vi "Error - Fire.vi"(8 "error in (no error)":errorcluster, 9 "Data":variant, 10 "Error Level":T6, 11 "View Model":T1) -> (0 "error out":errorcluster, 3 "View Model":T1)   [LabVIEW 2017]
doc: "Generates Error user event with parameters: Error Level, Error Data."
uses:
  View Model/Controls/View Model.ctl
  View Model/Controls/Shared Model.ctl
  Controls/Error Model.ctl
  Controls/Error Data.ctl
  Controls/Error Level.ctl
  Configuration/Controls/Config Model.ctl
  Configuration/Controls/Config Record.ctl
  Configuration/Controls/Config Data.ctl
  Configuration/Controls/Config Command.ctl
  Controller/Controls/Controler Model.ctl
  Views/Entry Console View/Controls/Entry Console - Wash Steps.ctl
  Controller/Controls/Controller - Overhead.ctl
  Controller/Controls/Controller - States.ctl
  Controller/Controls/Controller - Wash Step.ctl
  Views/Vehicle Position View/Controls/Vehicle - Station Enum.ctl
  Controller/Controls/Controller - Event.ctl
  Controller/Controls/Controller - Commands.ctl
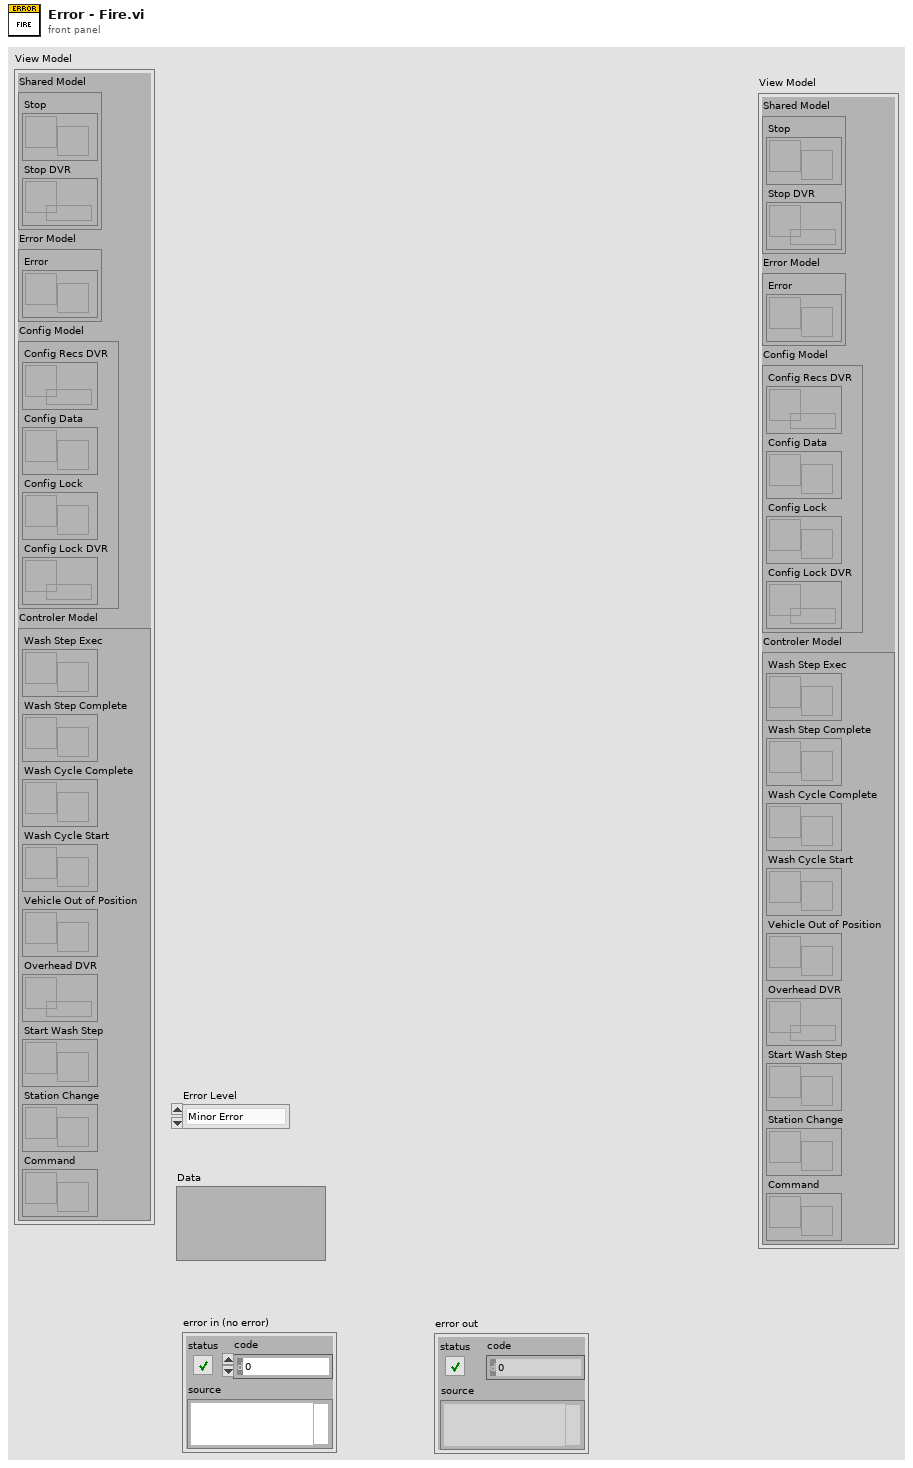
[diagram p1: front panel]
types:
  T1 = typedef "View Model.ctl" = cluster{"Shared Model":T2, "Error Model":T3, "Config Model":T4, "Controler Model":T5}
  T2 = typedef "Shared Model.ctl" = cluster{"Stop":refnum<user-event>, "Stop DVR":refnum<data-value>}
  T3 = typedef "Error Model.ctl" = cluster{"Error":refnum<user-event>}
  T4 = typedef "Config Model.ctl" = cluster{"Config Recs DVR":refnum<data-value>, "Config Data":refnum<user-event>, "Config Lock":refnum<user-event>, "Config Lock DVR":refnum<data-value>}
  T5 = typedef "Controler Model.ctl" = cluster{"Wash Step Exec":refnum<user-event>, "Wash Step Complete":refnum<user-event>, "Wash Cycle Complete":refnum<user-event>, "Wash Cycle Start":refnum<user-event>, "Vehicle Out of Position":refnum<user-event>, "Overhead DVR":refnum<data-value>, "Start Wash Step":refnum<user-event>, "Station Change":refnum<user-event>, "Command":refnum<user-event>}
  T6 = typedef "Error Level.ctl" = enum16{"Minor Error", "Wash Cycle Error", "System Error"}
  T7 = typedef "Error Data.ctl" = cluster{"Error Level":T6, "Data":variant}
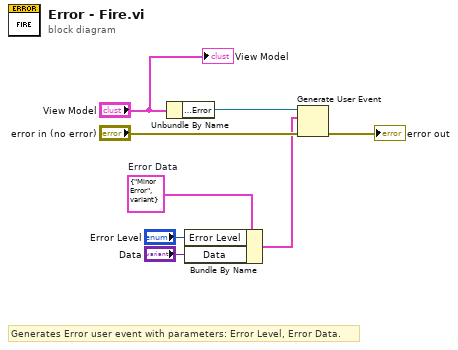
[diagram p0: block diagram]
diagram:
  w7 = T7 {"Error Level"=enum."Minor Error", "Data"=variant}  # Error Data
  # "Generates Error user event with parameters: Error Level, Error Data."
  n1 = Unbundle By Name("View Model") -> ("Error Model.Error"=w8:refnum<user-event>)
  n2 = Bundle By Name(cluster=w7, "Error Level"="Error Level", "Data"="Data") -> (w3:T7)
  n3 = Generate User Event(user event=w8, event data cluster=w3, error in="error in (no error)") -> (error out=→"error out":errorcluster)  [unwired: 1 in, 1 out]
  "View Model" <- "View Model"
